vi "DQMH_API_Init.vi"(0 "reference in":refnum<class "DQMH_API.lvclass"> caption="This control should only be used when\na sub class is inheriting this class", 11 "error in (no error)":errorcluster) -> (4 "reference out":refnum<class "DQMH_API.lvclass"> caption="This indicator should only be used when\na sub class is inheriting this class", 15 "error out":errorcluster)   [LabVIEW 2020, in "DQMH_API.lvclass"]
uses:
  <resource>/Framework/Providers/Open_GDS/UML/DQMH_API_class/DQMH_API.lvclass
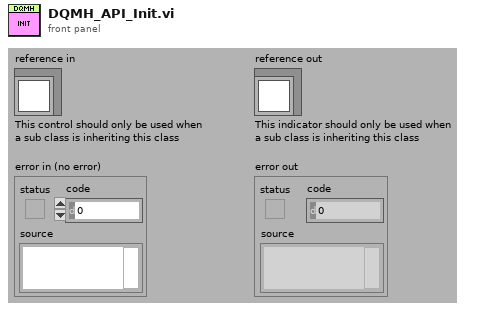
[diagram p1: front panel]
types:
  T1 = typedef "DQMH_API.lvclass/ObjectAttributes.ctl" = cluster{"Get Module Type Info":refnum<vi>, "Script New Module":refnum<vi>, "Script New Event":refnum<vi>, "Query Library for Module Info":refnum<vi>, "Parse Project for DQMH Modules":refnum<vi>, "Get All Events in Module":refnum<vi>}
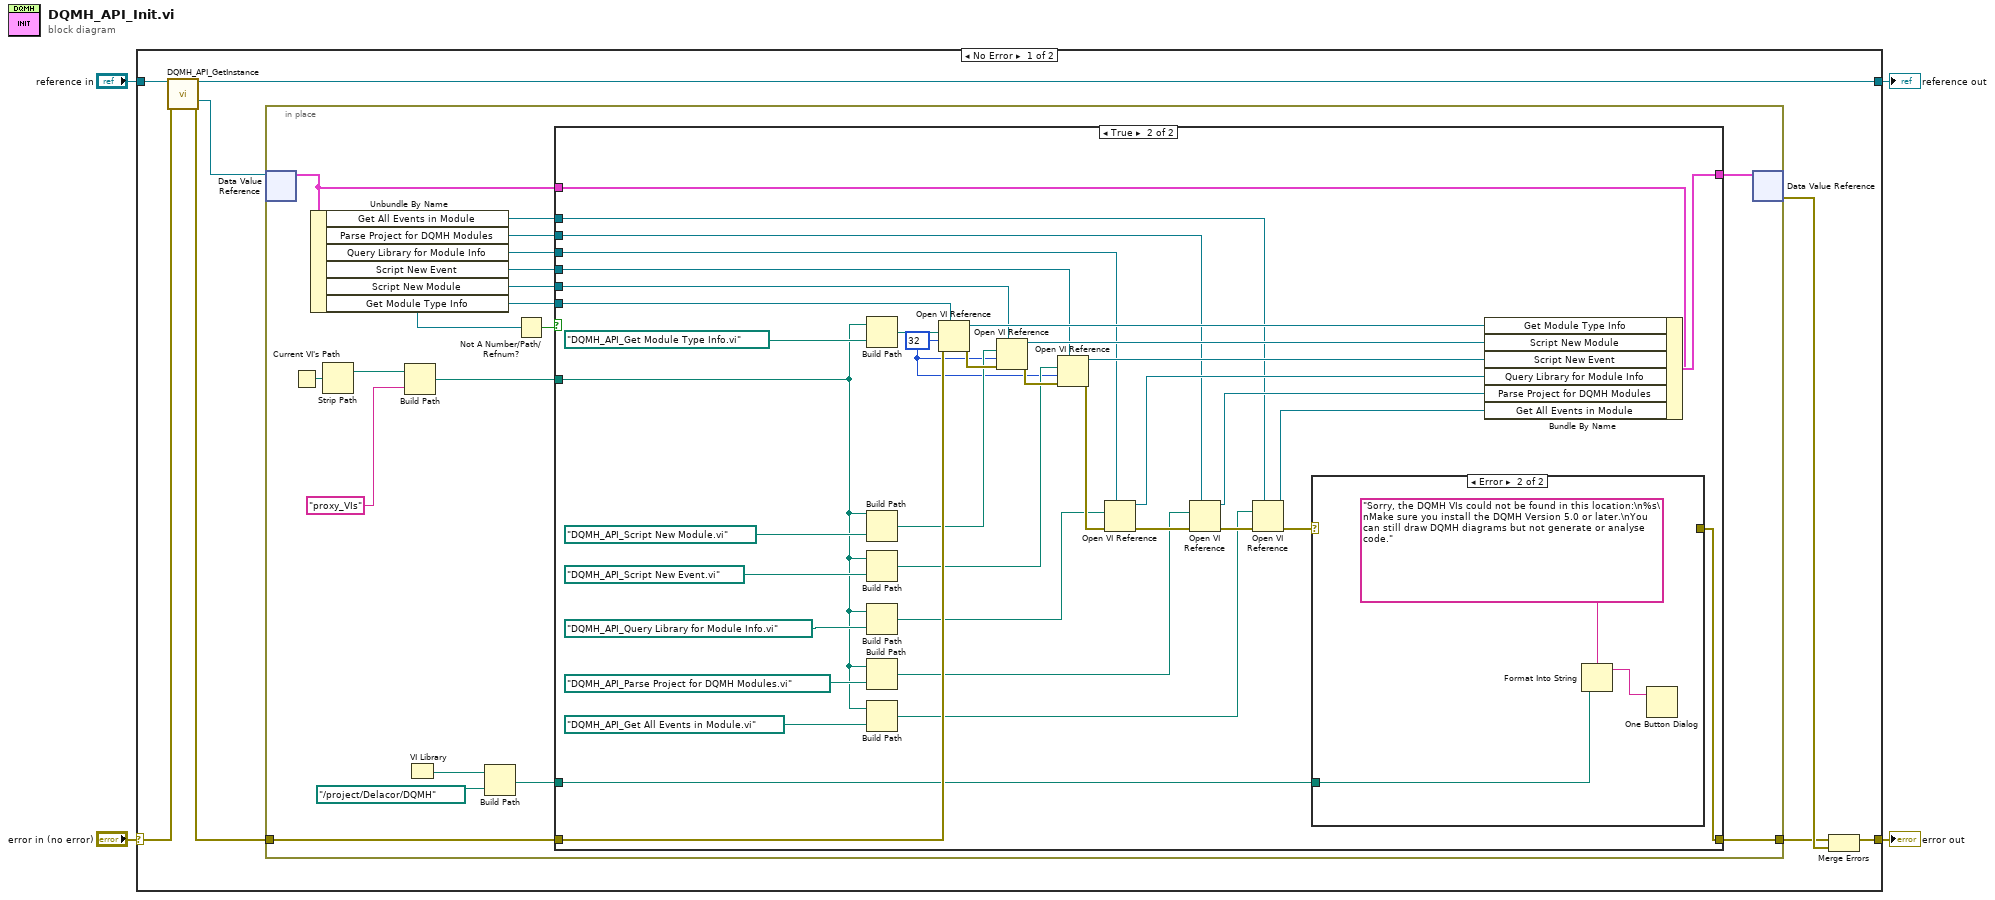
[diagram p0: block diagram]
diagram:
  n1 = case shown="No Error" "error in (no error)" {
    selector: "error in (no error)" -> [w10 w75]
    tunnel: [w11 w75] -> w3
    tunnel: "reference in" -> [w9 w74]
    tunnel: [w7 w74] -> w1
    frame No Error {
      n2 = call <resource>:"DQMH_API_GetInstance.vi"("reference in"=w9, "error in (no error)"=w10) -> ("reference out"=w7:refnum<class "DQMH_API.lvclass">, "DVRRefOut"=w8:refnum<data-value>, "error out"=w6:errorcluster)  [unwired: 9 in, 2 out]
      n3 = in-place {
        in-place-border: w6 -> [w27]
        in-place-border: [w26] -> w5
        n4 = in-place-dvr #1(w8) -> (w29:T1)  [unwired: 1 out]
        n5 = Current VI's Path() -> (path=w23:path)
        n6 = Unbundle By Name(w29) -> ("Get All Events in Module"=w13:refnum<vi>, "Parse Project for DQMH Modules"=w14:refnum<vi>, "Query Library for Module Info"=w16:refnum<vi>, "Script New Event"=w25:refnum<vi>, "Script New Module"=w28:refnum<vi>, "Get Module Type Info"=w15:refnum<vi>)
        n7 = Strip Path(path=w23) -> (stripped path=w22:path)  [unwired: 1 out]
        n8 = Build Path(base path=w22, name or relative path="proxy_VIs") -> (appended path=w20:path)
        n9 = VI Library() -> (path=w18:path)
        n10 = Build Path(base path=w18, name or relative path=path "../project/Delacor/DQMH" ("base path")) -> (appended path=w17:path)
        n11 = Not A Number/Path/Refnum?(number/path/refnum=w15) -> (NaN/Path/Refnum?=w24:bool)
        n12 = case shown="True" w24 {
          tunnel: [w32 w69] -> w30
          tunnel: w29 -> [w32 w68]
          tunnel: w28 -> [_ w58]
          tunnel: w27 -> [w31 w64]
          tunnel: [w31 w55] -> w26
          tunnel: w25 -> [_ w47]
          tunnel: w15 -> [_ w46]
          tunnel: w20 -> [_ w34]
          tunnel: w17 -> [_ w51]
          tunnel: w16 -> [_ w48]
          tunnel: w14 -> [_ w42]
          tunnel: w13 -> [_ w39]
          frame False {
          }
          frame True {
            w54 = 32 ("options")
            n13 = Build Path(base path=w34, name or relative path=path "DQMH_API_Get Module Type Info.vi") -> (appended path=w63:path)
            n14 = Build Path(base path=w34, name or relative path=path "DQMH_API_Script New Module.vi") -> (appended path=w57:path)
            n15 = Build Path(base path=w34, name or relative path=path "DQMH_API_Script New Event.vi") -> (appended path=w56:path)
            n16 = Build Path(base path=w34, name or relative path=path "DQMH_API_Query Library for Module Info.vi") -> (appended path=w50:path)
            n17 = Build Path(base path=w34, name or relative path=path "DQMH_API_Parse Project for DQMH Modules.vi") -> (appended path=w43:path)
            n18 = Build Path(base path=w34, name or relative path=path "DQMH_API_Get All Events in Module.vi") -> (appended path=w36:path)
            n19 = Open VI Reference(type specifier VI Refnum (for type only)=w46, vi path=w63, options=w54, error in (no error)=w64) -> (vi reference=w67:refnum<vi>, error out=w66:errorcluster)  [unwired: 2 in]
            n20 = Open VI Reference(type specifier VI Refnum (for type only)=w58, vi path=w57, options=w54, error in (no error)=w66) -> (vi reference=w65:refnum<vi>, error out=w60:errorcluster)  [unwired: 2 in]
            n21 = Open VI Reference(type specifier VI Refnum (for type only)=w47, vi path=w56, options=w54, error in (no error)=w60) -> (vi reference=w59:refnum<vi>, error out=w52:errorcluster)  [unwired: 2 in]
            n22 = Open VI Reference(type specifier VI Refnum (for type only)=w48, vi path=w50, error in (no error)=w52) -> (vi reference=w49:refnum<vi>, error out=w45:errorcluster)  [unwired: 3 in]
            n23 = Open VI Reference(type specifier VI Refnum (for type only)=w42, vi path=w43, error in (no error)=w45) -> (vi reference=w41:refnum<vi>, error out=w40:errorcluster)  [unwired: 3 in]
            n24 = Open VI Reference(type specifier VI Refnum (for type only)=w39, vi path=w36, error in (no error)=w40) -> (vi reference=w38:refnum<vi>, error out=w33:errorcluster)  [unwired: 3 in]
            n25 = case shown="Error" w33 {
              selector: w33 -> [w70 _]
              tunnel: [w70 _] -> w55
              tunnel: w51 -> [_ w71]
              frame No Error {
              }
              frame Error {
                n26 = Format Into String(format string="Sorry, the DQMH VIs could not be found in this location:\n%s\nMake sure you install the DQMH Version 5.0 or later.\nYou can still draw DQMH diagrams but not generate or analyse code.", w71) -> (resulting string=w72:string)  [unwired: 2 in, 1 out]
                n27 = One Button Dialog(message=w72) -> ()  [unwired: 1 in, 1 out]
              }
            }
            n28 = Bundle By Name(cluster=w68, "Get Module Type Info"=w67, "Script New Module"=w65, "Script New Event"=w59, "Query Library for Module Info"=w49, "Parse Project for DQMH Modules"=w41, "Get All Events in Module"=w38) -> (w69:T1)
          }
        }
        n29 = in-place-dvr #1(w30) -> (w12:errorcluster)  [unwired: 1 out]
      }
      n30 = Merge Errors(w5, w12) -> (w11:errorcluster)
    }
    frame Error {
    }
  }
  "error out" <- w3
  "reference out" <- w1
